vi "WPI_IMU_ADIS16460_WriteCommand.vi"(8 "error in (no error)":errorcluster, 9 "Data":u16=2049, 10 "ADIS16460 Register":T1=62 items=["PROD_ID"=86, "GLOB_CMD"=62, "DEC_RATE"=54, "FLTR_CTRL"=56, "MSC_CTRL"=50], 11 "SPIDevRef in":T2) -> (0 "error out":errorcluster, 3 "SPIDevRef out":T2)   [LabVIEW 2015, in "FRC ADIS16460.lvlib"]
uses:
  FRC ADIS16460.lvlib
  <vilib>/Rock Robotics/SystemInterfaces/spilib/spi_bus.ctl
  <vilib>/Rock Robotics/WPI/SPI/WPI_SPIDevRef.ctl
  WPI_IMU_ADIS16460_Registers.ctl
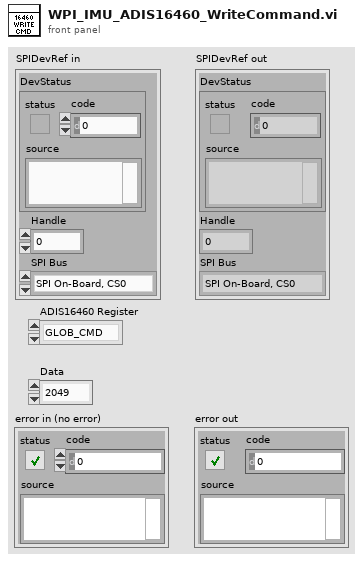
[diagram p1: front panel]
types:
  T1 = typedef "FRC ADIS16460.lvlib/WPI_IMU_ADIS16460_Registers.ctl" = u8
  T2 = typedef "WPI_SPIDevRef.ctl" = cluster{"DevStatus":errorcluster, "Handle":i32, "SPI Bus":T3}
  T3 = typedef "spi_bus.ctl" = enum16{"SPI On-Board, CS0", "SPI On-Board, CS1", "SPI On-Board, CS2", "SPI On-Board, CS3", "SPI MXP", "Invalid"}
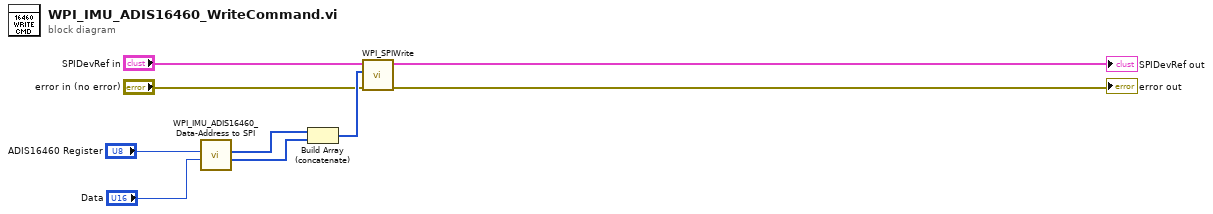
[diagram p0: block diagram]
diagram:
  n1 = call "WPI_IMU_ADIS16460_Data-Address to SPI.vi"("Data"="Data", "Address"="ADIS16460 Register") -> ("Low Word"=w7:u8[], "High Word"=w8:u8[])  [unwired: 8 in]
  n2 = Build Array (concatenate)(w8, w7) -> (w9:u8[])
  n3 = call <vilib>:"WPI_SPIWrite.vi"("error in (no error)"="error in (no error)", "Data To Send"=w9, "SPIDevRef"="SPIDevRef in") -> ("error out"=→"error out":errorcluster, "SPIDevRef"=→"SPIDevRef out":T2)  [unwired: 7 out]
